vi "Stop Core.vi"(10 "final error code":i32, 11 "Template in":refnum<class "Template.lvclass">) -> (3 "Template out":refnum<class "Template.lvclass">)   [LabVIEW 2020, in "Template.lvlib" / "Template.lvclass"]
doc: "(<B>Filename</B>: Actor Framework.lvlib:Actor.lvclass:Stop Core.vi)\n\nDefines what the actor does before it stops. Use the <B>final error code</B> input to determine whether the actor shut down in response to an error.\n\nBy default, this method passes the Stop message along to all auto-stop nested actors. A descendant class may override this method to define additional behavior, such as shutting down any processes the actor initiated in its override of the Actor Core method."
uses:
  Template.lvclass
  Template.lvclass/Template.ctl
  <vilib>/ActorFramework/Actor/Actor.lvclass
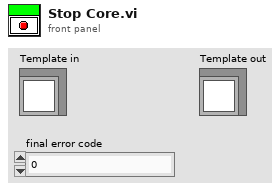
[diagram p1: front panel]
types:
  T1 = typedef "Template.lvlib/Template.lvclass/actor configuration.ctl" = cluster{"GlobalConfiguration":T2, "DeviceConfiguration":T3}
  T2 = typedef "Template.lvlib/Template.lvclass/shared actor configuration.ctl" = cluster{"DeviceFamily":string, "WriteData":bool, "BufferSize_samples":i32, "SyncDevice":bool, "ExecuteInterruptRoutine":bool, "InterruptRoutineTimeout_ms":i32}
  T3 = typedef "Template.lvlib/Template.lvclass/device configuration cluster.ctl" = cluster{"DeviceSpecificName":string, "HardwareReference":string, "UsedResources":T4[]}
  T4 = typedef "Template.lvlib/Template.lvclass/single resource cluster.ctl" = cluster{"ResourceLocation":string, "ResourceData":variant}
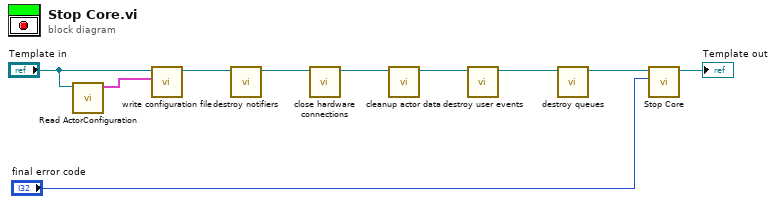
[diagram p0: block diagram]
diagram:
  n1 = call "Read ActorConfiguration.vi"("Template in"="Template in") -> ("ActorConfiguration"=w5:T1)  [unwired: 10 in]
  n2 = call-dynamic "write configuration file.vi"("ActorConfiguration"=w5, "Template in"="Template in") -> ("Template out"=w3:refnum<class "Template.lvclass">)  [unwired: 9 in]
  n3 = call-dynamic "destroy notifiers.vi"("Template in"=w3) -> ("Template out"=w2:refnum<class "Template.lvclass">)  [unwired: 10 in]
  n4 = call-dynamic "close hardware connections.vi"("Template in"=w2) -> ("Template out"=w8:refnum<class "Template.lvclass">)  [unwired: 10 in]
  n5 = call-dynamic "cleanup actor data.vi"("Template in"=w8) -> ("Template out"=w7:refnum<class "Template.lvclass">)  [unwired: 10 in]
  n6 = call-dynamic "destroy user events.vi"("Template in"=w7) -> ("Template out"=w6:refnum<class "Template.lvclass">)  [unwired: 10 in]
  n7 = call-dynamic "destroy queues.vi"("Template in"=w6) -> ("Template out"=w1:refnum<class "Template.lvclass">)  [unwired: 10 in]
  n8 = call-parent "Stop Core.vi"("final error code"="final error code", "Actor in"=w1) -> ("Actor out"=→"Template out":refnum<class "Template.lvclass">)  [unwired: 9 in]
